vi "_TangoSetTimeout.vi"(1 "error in":errorcluster, 2 "tmo_in_msecs":u32, 3 "device_name":string) -> (0 "error out":errorcluster)   [LabVIEW 2014, in "tango.lvlib"]
uses:
  tango.lvlib
  tango_binding.so
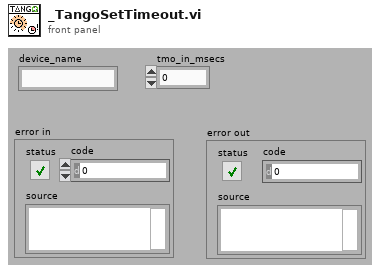
[diagram p1: front panel]
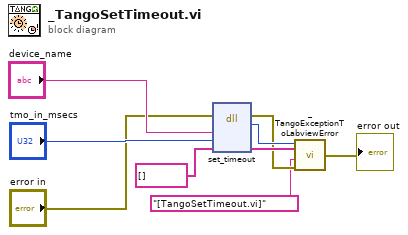
[diagram p0: block diagram]
diagram:
  n1 = dll-call lib="tango_binding.*" fn="set_timeout"(error in="error in", "device_name"="device_name", "tmo_in_msecs"="tmo_in_msecs", "error_stack"=string[] [] ("error stack")) -> (error out=w3:errorcluster, "return type"=w5:i32, "error_stack"=w4:string[])  [unwired: 4 in, 1 out]
  n2 = call "_TangoExceptionToLabviewError.vi"("error in"=w3, "location"="[TangoSetTimeout.vi]", "error stack"=w4, "error code"=w5) -> ("error out"=→"error out":errorcluster)
